vi "ASIC_WRITE_CHECK.vi"(0 "ftHandle_in":u32, 1 "Direccion Registro Asic":u8, 2 "Byte Alto":u8, 3 "Byte Bajo":u8, 5 "error in":errorcluster, 6 "Espera acceso USB 2":u32) -> (14 "ftHandle_out":u32, 15 "Write OK":bool, 19 "error out":errorcluster)   [LabVIEW 2019]
uses:
  Global cuenta erroes.vi
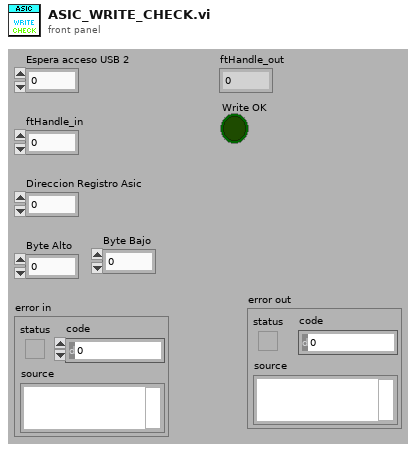
[diagram p1: front panel]
types:
  T1 = typedef "global erroes cluster.ctl" = cluster{"Errores FPGA":i32, "Errores Asic":i32, "Errores ADC adq":i32, "Errores ADC Asic":i32}
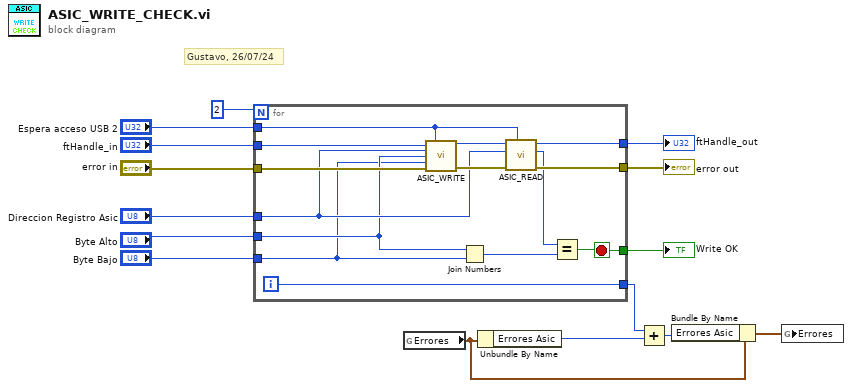
[diagram p0: block diagram]
diagram:
  # "Gustavo, 26/07/24"
  n1 = for {
    N: 2 -> [_]
    tunnel: "Espera acceso USB 2" -> [w27]
    tunnel: [w26] -> w8
    tunnel: [w25] -> w9
    tunnel: "ftHandle_in" -> [w24]
    tunnel: "error in" -> [w23]
    tunnel: "Direccion Registro Asic" -> [w22]
    tunnel: "Byte Alto" -> [w20]
    tunnel: "Byte Bajo" -> [w19]
    tunnel: [w17] -> w6
    tunnel: [w16] -> w5
    i -> [w16]
    stop <- w17 stop-if-true
    n2 = call "ASIC_WRITE.vi"("ftHandle_in"=w24, "Espera acceso USB"=w27, "Direccion Registro Asic"=w22, "Byte Alto"=w20, "Byte Bajo"=w19, "error in"=w23) -> ("ftHandle_out"=w29:u32, "error out"=w28:errorcluster)  [unwired: 8 in]
    n3 = Join Numbers(hi=w20, lo=w19) -> ((hi.lo)=w18:u16)
    n4 = call "ASIC_READ.vi"("Espera acceso USB"=w27, "error in"=w28, "Direccion Registro Asic"=w22, "ftHandle_in"=w29) -> ("error out"=w25:errorcluster, "Valor Asic"=w21:u16, "ftHandle_out"=w26:u32)  [unwired: 5 in]
    n5 = Equal?(x=w21, y=w18) -> (x = y?=w17:bool)
  }
  "error out" <- w9
  "ftHandle_out" <- w8
  "Write OK" <- w6
  n6 = global read "Global cuenta erroes.vi" "Errores"() -> (w3:T1)
  n7 = Unbundle By Name(w3) -> ("Errores Asic"=w4:i32)
  n8 = Add(x=w5, y=w4) -> (x+y=w1:i32)
  n9 = Bundle By Name(cluster=w3, "Errores Asic"=w1) -> (w2:T1)
  n10 = global write "Global cuenta erroes.vi" "Errores"(w2) -> ()
